vi "DAQ Status.vi"(7 "Enum":T1, 11 "Async_Status":T2) -> (2 "DAQ Error?":bool, 3 "Valid":bool)   [LabVIEW 2015]
uses:
  ATS-VI/ATS_ctl/ATS_Async_Status.ctl
  DAQ Status States.ctl
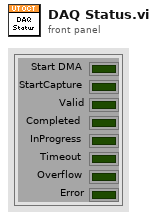
[diagram p1: front panel]
types:
  T1 = typedef "DAQ Status States.ctl" = enum16{"Get", "Show"}
  T2 = typedef "ATS_Async_Status.ctl" = cluster{"Start DMA":bool, "StartCapture":bool, "Valid":bool, "Completed":bool, "InProgress":bool, "Timeout":bool, "Overflow":bool, "Error":bool}
  T3 = enum32{"Invalid", "Standard", "Closed", "Hidden", "Minimized", "Maximized"}
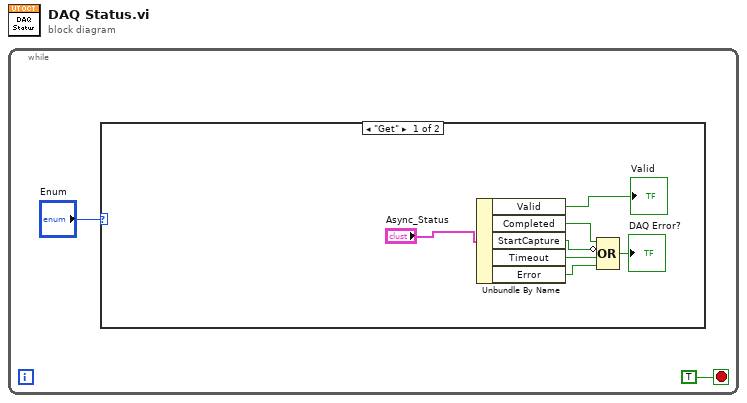
[diagram p0: block diagram]
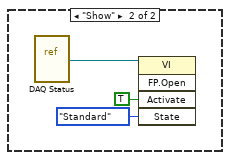
[diagram p2: hidden frame]
diagram:
  n1 = while {
    stop <- TRUE stop-if-true
    n2 = case shown="\"Get\"" "Enum" {
      frame "Get" {
        n3 = Unbundle By Name("Async_Status") -> ("Valid"=→"Valid":bool, "Completed"=w6:bool, "StartCapture"=w7:bool, "Timeout"=w9:bool, "Error"=w8:bool)
        n4 = Compound Arithmetic op=OR(w6, invert w7, w9, w8) -> (→"DAQ Error?":bool)
      }
      frame "Show" {
        n5 = vi-ref "DAQ Status.vi"() -> (w12:refnum<vi>)
        n6 = invoke class="VI" method="FP.Open"(reference=w12, "Activate"=TRUE ("Activate?"), "State"=T3."Standard") -> ()  [unwired: 2 in, 5 out]
      }
    }
  }
